vi "Sync.vi"(8 "error in (no error)":errorcluster, 10 "timeout in ms (-1)":i32, 11 "DAQmx-Bus in":refnum<class "DAQmx-Bus.lvclass">) -> (0 "error out":errorcluster, 2 "timed out?":bool, 3 "DAQmx-Bus out":refnum<class "DAQmx-Bus.lvclass">)   [LabVIEW 2021, in "DAQmx-Bus.lvclass"]
uses:
  DAQmx-Bus.lvclass
  DAQmx-Bus.lvclass/DAQmx-Bus.ctl
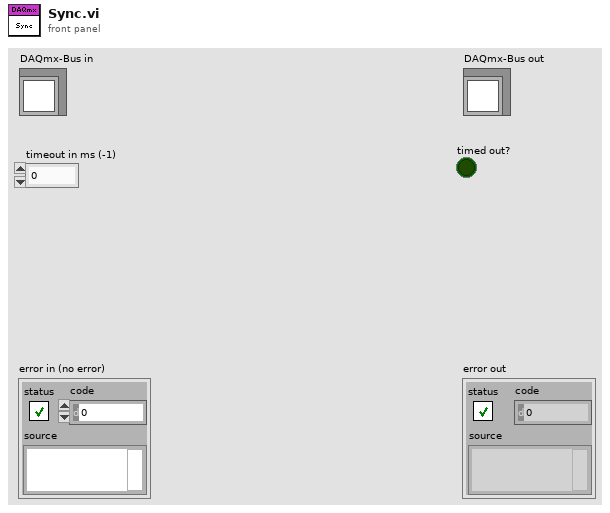
[diagram p1: front panel]
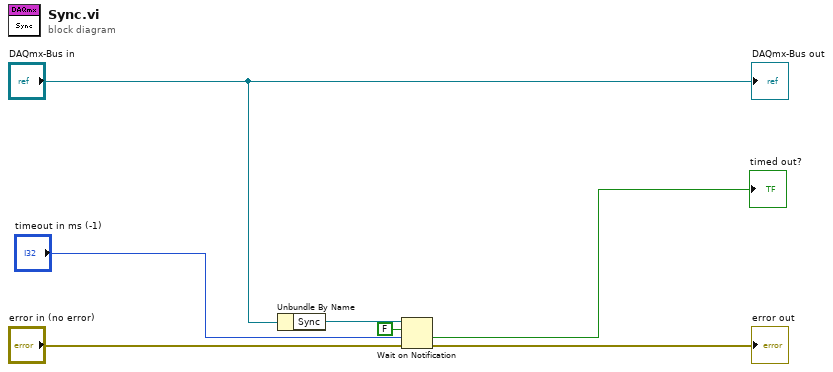
[diagram p0: block diagram]
diagram:
  n1 = Unbundle By Name("DAQmx-Bus in") -> ("Sync"=w4:refnum<notifier>)
  n2 = Wait on Notification(notifier=w4, ignore previous (F)=FALSE, timeout in ms (-1)="timeout in ms (-1)", error in (no error)="error in (no error)") -> (timed out?=→"timed out?":bool, error out=→"error out":errorcluster)  [unwired: 2 out]
  "DAQmx-Bus out" <- "DAQmx-Bus in"
